vi "AlliGator Update Loaded Dataset Info.vi"(4 "Image Loading Options":T1={"Pixel Well Capacity"=0, "Pile-up Correction"=FALSE, "Gate Step"=0, "Image Smoothing Options"={"Use Image Smoothing"=FALSE, "Kernel Type"=enum."Bilinear", "Bin"=1, "Algorithm"=enum."Rapid"}, "Gates to Skip"={"Start"=0, "End"=0}, "File Background Subtraction"=FALSE, "Background File Path"=path "", "Image Binning Options"={"Use Image Binning"=FALSE, "X Bin"=1, "Y Bin"=1}, "# Gates"=0, "Gates to Keep"={"First"=0, "Last"=0}, "Define Gates to"=FALSE, "Hot Pixel Removal"={"Remove Screamers"=FALSE, "Delta"=0.0, "Equalize Histogram"=FALSE, "Percentile"=0.0, "Hot Pixel Mask Image"=path "", "Use Hot Pixel Mask"=FALSE}, "Dataset Scaling Factor"=0.0, "Image Pre-processing Steps"=[]} {"Hot Pixel Removal"."Percentile" min=0 max=100; "Image Binning Options"."Y Bin" min=1; "Image Binning Options"."X Bin" min=1; "Image Smoothing Options"."Bin" min=1}, 6 "Background File?":bool, 7 "Pile-up Correction":bool, 8 "error in (no error)":errorcluster, 9 "After Loading Dataset Information":T10, 10 "# Gates":i32, 11 "Pixel Well Capacity":u32) -> (0 "Error Out":errorcluster)   [LabVIEW 2021, in "AlliGator Files.lvlib"]
doc: "Updates Settings and Internal Variables after loading a new dataset."
uses:
  AlliGator Files.lvlib
  AlliGator After Loading Dataset Information.ctl
  AlliGator ICCD-specific Information.ctl
  Source Image/AlliGator Image Loading Options.ctl
  Settings/AlliGator Image Smoothing Options.ctl
  Arrays/Kernel Type.ctl
  Arrays/Smoothing Algorithm.ctl
  Settings/AlliGator Background Subtraction Parameters.ctl
  Source Image/AlliGator Image Binning Options.ctl
  Settings/AlliGator Gates to Keep.ctl
  SwissSPAD/SwissSPAD Live_Image Display Options.ctl
  AlliGator Image Pre-processing Step.ctl
  Globals, Variables, Constants/AlliGator Variables List.ctl
  Settings/AlliGator Settings List.ctl
  Globals, Variables, Constants/AlliGator Refnums List.ctl
  Globals, Variables, Constants/AlliGator Globals, Variables & Constants.lvlib
  Settings/AlliGator Settings.lvlib
  GUI/AlliGator GUI.lvlib
  Arrays/Arrays.lvlib
  Source Image/AlliGator Source Image.lvlib
  SwissSPAD/SwissSPAD Live.lvlib
panel:
  # "see the AlliGator License on the block diagram (Ctrl+E or Window:Show Block Diagram)"
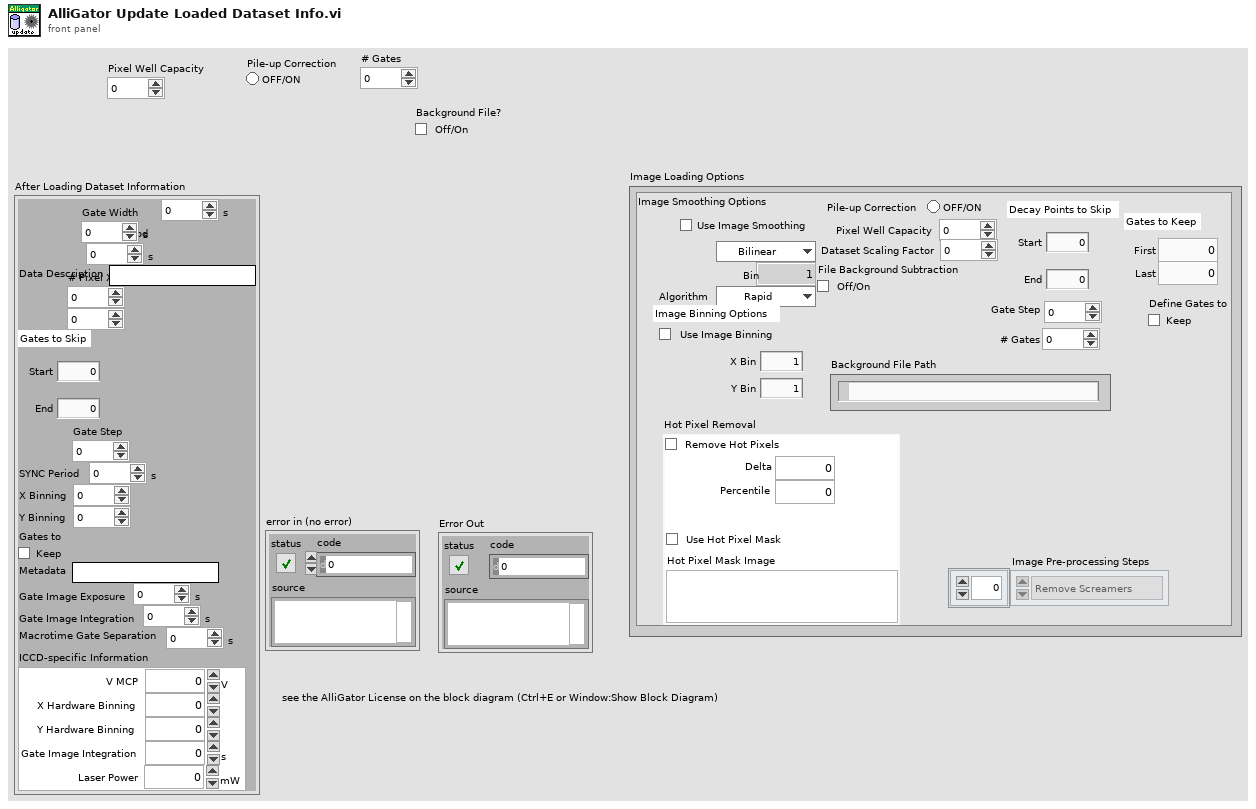
[diagram p1: front panel]
types:
  T1 = typedef "AlliGator Source Image.lvlib/AlliGator Image Loading Options.ctl" = cluster{"Pixel Well Capacity":u32, "Pile-up Correction":bool, "Gate Step":i32, "Image Smoothing Options":T2, "Gates to Skip":T5, "File Background Subtraction":bool, "Background File Path":path, "Image Binning Options":T6, "# Gates":u32, "Gates to Keep":T7, "Define Gates to":bool, "Hot Pixel Removal":T8, "Dataset Scaling Factor":dbl, "Image Pre-processing Steps":T9[]}
  T2 = typedef "AlliGator Settings.lvlib/AlliGator Image Smoothing Options.ctl" = cluster{"Use Image Smoothing":bool, "Kernel Type":T3, "Bin":i32, "Algorithm":T4}
  T3 = typedef "Arrays.lvlib/Kernel Type.ctl" = enum16{"Uniform", "Bilinear", "Gaussian"}
  T4 = typedef "Arrays.lvlib/Smoothing Algorithm.ctl" = enum16{"Rapid", "Thorough"}
  T5 = typedef "AlliGator Settings.lvlib/AlliGator Background Subtraction Parameters.ctl" = cluster{"Start":u32, "End":u32}
  T6 = typedef "AlliGator Source Image.lvlib/AlliGator Image Binning Options.ctl" = cluster{"Use Image Binning":bool, "X Bin":i32, "Y Bin":i32}
  T7 = typedef "AlliGator Settings.lvlib/AlliGator Gates to Keep.ctl" = cluster{"First":u32, "Last":u32}
  T8 = typedef "SwissSPAD Live.lvlib/SwissSPAD Live_Image Display Options.ctl" = cluster{"Remove Screamers":bool, "Delta":sgl, "Equalize Histogram":bool, "Percentile":sgl, "Hot Pixel Mask Image":path, "Use Hot Pixel Mask":bool}
  T9 = typedef "AlliGator Files.lvlib/AlliGator Image Pre-processing Step.ctl" = enum16{"Remove Screamers", "Pile-up Correction", "Binning", "Smoothing", "Rescaling", "Dead Left Column Correction"}
  T10 = typedef "AlliGator Files.lvlib/AlliGator After Loading Dataset Information.ctl" = cluster{"Nanotime Gate Separation":dbl[unit], "Gate Width":dbl[unit], "Laser Period":dbl[unit], "Data Description":string, "# Pixel X":i32, "# Pixel Y":i32, "Gates to Use":cluster{"Start":u32, "End":u32}, "Gate Step":i32, "SYNC Period":dbl[unit], "X Binning":i32, "Y Binning":i32, "Gates to":bool, "Metadata":string, "Gate Image Exposure":dbl[unit], "Gate Image Integration":dbl[unit], "Macrotime Gate Separation":dbl[unit], "ICCD-specific Information":T11}
  T11 = typedef "AlliGator Files.lvlib/AlliGator ICCD-specific Information.ctl" = cluster{"V MCP":dbl[unit], "X Hardware Binning":dbl, "Y Hardware Binning":dbl, "Gate Image Integration":dbl[unit], "Laser Power":dbl[unit]}
  T12 = typedef "AlliGator Globals, Variables & Constants.lvlib/AlliGator Variables List.ctl" = enum16{"---- GUI ----", "GUI:Initialization Status", "GUI:State Indicators Refnum", "GUI:Original AlliGator Menu Items", "GUI:Current Action Loop State", "GUI:Script in progress", "GUI:Playback", "GUI:Loop Playback", "GUI:Search ROI Used", "GUI:Search ROI", "Decay Graph Max Legend Size", "Intensity Graph Max Legend Size", "Decay Statistics Graph Max Legend Size", "Phasor Graph Max Legend Size", "Phasor Ratio Graph Max Legend Size", "Lifetime Graph Max Legend Size", "---- Files ----", "Files:Export Dataset Frames as Individual Files", "Files:Show Batch Export Help Balloons", "Files:Frames in Dataset", "Files:ptu File Frame Start Indices", "Files:Current Frame in Dataset", "Files:Current Frame Timestamp", "Files:Dataset Loaded", "Files:Dataset Metadata", "Files:Dataset Channel", "Files:Dataset Data Description", "Files:Background Dataset Metadata", "Files:Background Dataset Channel", "Files:Background Dataset Data Description", "Files:Background File Subtraction", "Files:Background File Path", "Files:Background File Pile-up Correction", "Files:Background File Pixel Well Capacity", "Files:Background File Scaling Factor", "Files:Current Dataset Load Settings", "Files:Dataset Path", "Files:ICCD-specific Information", "Files:Macrotime Gate Separation", "------ Python Plugins ------", "Python Plugins:Information", "Python Plugins:Python Session", "Python Plugins:Valid Python Session?", "---- Source Image ----", "Source Image:ROIs", "Source Image:Current ROI", "Source Image:ROI Event Refnum", "X_Source Image Display Range", "X_Source Image Palette Information", "X_Type of Displayed Image", "X_Time Gate Slider", "Source Image:Palette List", "Source Image:Scale", "Source Image:ROI Overlay Color", "Source Image:Overlay to Erase", "Source Image:Is Displayed Image Accumulated", "Source Image:White Light Image Modified", "Source Image:Mask Image Modified", "---- Image Profile Window ----", "Image Profile:Window Event Refnum", "Image Profile:IntensityType", "Image Profile:Intensity Average Type", "Image Profile:Intensity-weighted SDV", "Image Profile:Box Profile Type", "Image Profile:Window Open", "Image Profile:Plotted Fit Parameter", "------ Phasor Graph -------", "Phasor Graph:Show Line", "---- Phasor Plot ---", "Phasor Plot:Parameters Changed", "Phasor Plot:FLI Dataset Modified since last Calculation", "Phasor Harmonics Data", "Selected Phasor Harmonics", "Phasor Harmonic Manager Event Refnum", "Phasor Plot:ROIs", "Phasor Plot:Current ROI", "Phasor Plot:ROI Event Refnum", "Phasor Plot:Image Reference Points", "Phasor Plot:Computed", "Phasor Plot:Palette Information", "Phasor Plot:Palette List", "Phasor Plot:Phasor Ratio Palette Information", "Phasor Plot:Phasor Ratio Palette List", "Phasor Plot:Image Scale", "Phasor Plot:Image Overlay to Erase", "Phasor Plot:Image Elements to Update", "Phasor Plot:Current Calculation Parameters", "Phasor Plot:Current Calibration Options", "Phasor Plot:Reset Cumulated Phasor Plot", "Phasor Plot:Reference 1", "Phasor Plot:Lifetime Reference 1", "Phasor Plot:Reference 1 Frequency", "Phasor Plot:Reference 2", "Phasor Plot:Lifetime Reference 2", "Phasor Plot:Reference 2 Frequency", "---- Decay Analysis ----", "Number of Selected Decays to Fit", "LS Fit Results", "LAR Fit Results", "BS Fit Results", "Last Decay Max - Min", "Best Fit Parameters", "Best Fit Parameter Names", "Actual Size X", "Actual Size Y", "Binning X", "Binning Y", "Actual # Gates", "Dataset Number", "Gates to...", "Gates Skipped", "Gates to keep", "Gate Step", "Gate Separation", "Reversed Gates", "Pile-up Correction", "Pixel Well Capacity", "Background Subtracted", "Background Subtraction Method", "Background Definition Range", "Background File (deprecated)", "Number of Dataset Accumulated", "Array of Accumulated Dataset Paths", "Do Averaged Datasets", "Destination File Path", "Process Plot Target", "Use 1/D as Phasor Frequency", "---- Decay Fit Parameter Map -----", "Decay Fit Parameter Map:Palette Information", "Decay Fit Parameter Map:Palette List", "---- Parameter Map ----", "Parameter Map:Palette Information", "Parameter Map:Palette List", "------- Local Decay Window ---------", "Local Decay Graph Window:Event Refnum", "Local Decay Graph Window:Use normalized IRF for convolution", "----- Miscellaneous ----", "Misc:Skippable Dialog Windows Status"}
  T13 = typedef "AlliGator Settings.lvlib/AlliGator Settings List.ctl" = enum16{"GUI:Visible Settings Tab", "GUI:Last Run Version", "Source Image:Use Image Histogram for Contrast", "Source Image:Low Count Pixels Rejection Options", "Source Image:High Count Pixels Rejection Options", "Source Image:Use Image Brightness", "Source Image:Blend Overlay with Image Background", "Source Image:Use Fixed ROI Diameter", "Source Image:ROI Diameter", "Source Image:ROI Center Color", "Source Image:Peak Threshold", "Source Image:Intensity Threshold", "Source Image:Image Binning Options", "Source Image:Image Smoothing Options", "Source Image:Image Histogram Active", "Source Image:Invert Binary Mask", "Source Image:Hot Pixel Removal", "Source Image:Overlay Analyzed ROI Center", "Source Image:Auto-Adjust Contrast", "Source Image:Histogram Lower Percentile", "Source Image:Histogram Upper Percentile", "Source Image:Save Source Image", "Source Image:Scale Bar Options", "Source Image:Image Resolution (Pixel Size)", "Source Image:Flatfield Correction", "Source Image:Show Dead Left Columns Correction", "Source Image:Dead Left Columns Correction", "Source Image:Image Pre-Processing Operations Order", "Source Image:Overlay ROI Median", "Source Image:Median Overlay Color", "Data Information:Gate Width", "Data Information:Nanotime Gate Separation", "Data Information:Macrotime Gate Separation", "Data Information:Gate Step", "Data Information:# Gates", "Data Information:Gate Image Exposure", "Data Information:Gate Image Integration", "Data Information:Gates to Skip", "Data Information:Gates to Keep", "Data Information:Define Gates to", "Data Information:Channel Name", "Data Information:Available Channel Names", "Data Information:Channel Arithmetic", "Data Information:Background File Subtraction", "Data Information:Background File", "Data Information:Background Scaling Factor", "Data Information:Background Pile-up Correction", "Data Information:Background Pixel Well Capacity", "Data Information:Laser Period", "Data Information:SYNC Period", "Data Information:Pile-up Correction", "Data Information:Pixel Well Capacity", "Data Information:Dataset Scaling Factor", "Fluorescence Decay_Decay Pre-Processing:Reverse Gates", "Fluorescence Decay_Decay Pre-Processing:Verbose Decay Pre-Processing", "Fluorescence Decay_Decay Pre-Processing:Use Decay Pre-Processing", "Fluorescence Decay_Decay Pre-Processing:Background Subtraction", "Fluorescence Decay_Decay Pre-Processing:Background Definition Range", "Fluorescence Decay_Decay Pre-Processing:Baseline Subtraction Method", "Fluorescence Decay_Decay Pre-Processing:Decay Pre-Processing Operations Order", "Fluorescence Decay_Decay Pre-Processing:Smoothing Parameter", "Fluorescence Decay_Decay Pre-Processing:Shift Decay", "Fluorescence Decay_Decay Pre-Processing:Decay Shift Parameters", "Fluorescence Decay_Decay Pre-Processing:Fold Decay", "Fluorescence Decay_Decay Pre-Processing:# Folds", "Fluorescence Decay_Decay Pre-Processing:1-Normalize Decay", "Fluorescence Decay_Decay Pre-Processing:[0-1]-Normalize Decay", "Fluorescence Decay_Decay Pre-Processing:Smoothen Decay", "Fluorescence Decay_Decay Pre-Processing:Extrapolate Decay", "Fluorescence Decay_Decay Pre-Processing:Use Periodicity", "Fluorescence Decay_Decay Pre-Processing:Use Cursors", "Fluorescence Decay_Decay Pre-Processing:Tail Fraction", "Fluorescence Decay_Decay Pre-Processing:Head Fraction", "Fluorescence Decay_Decay Pre-Processing:Additional Points", "Fluorescence Decay_Decay Pre-Processing:Straighten Decay", "Fluorescence Decay_Decay Pre-Processing:Constant Background", "Fluorescence Decay_Decay Pre-Processing:Pixel-Normalize Decay", "Fluorescence Decay_Advanced Analysis:Extract IRF instead of Decay", "Fluorescence Decay_Advanced Analysis:IRF Extraction Options", "Fluorescence Decay_Advanced Analysis:IRF Optimization Options", "Fluorescence Decay_Advanced Analysis:Square Pulse Options", "Fluorescence Decay_Advanced Analysis:IRF Order", "Fluorescence Decay_Advanced Analysis:IRF Time Constants", "Fluorescence Decay_Advanced Analysis:Wavelet Analysis Options", "Fluorescence Decay_Advanced Analysis:Average Lifetime Options", "Fluorescence Decay_Fit Options:Fit Options", "Fluorescence Decay_Fit Options:Use Legacy Fitting Approach", "Fluorescence Decay_Fit Options:Use Data Information Laser Period", "Fluorescence Decay_Fit Parameters:Displayed Fit Parameters", "Fluorescence Decay_Fit Parameters:Fit Parameter Constraints", "Fluorescence Decay_Fit Parameters:Export Tabulated Results", "Fluorescence Decay_Fit Parameters:MLE Baseline Offset Type", "Fluorescence Decay_Fit Parameters:MLE Baseline Offset", "Fluorescence Decay_Fit Parameters:Guess Parameter Names", "Fluorescence Decay_Fit Parameters:Guess Parameter Values", "Fluorescence Decay_Fit Parameters:Guess Parameters Options", "Fluorescence Decay_Styles:Show Last Decay Only", "Fluorescence Decay_Styles:Decay Graph Color Array", "Fluorescence Decay:Decay Graph Active", "Fluorescence Decay Statistics:Min Peak Value", "Fluorescence Decay Statistics:Reject Low Decay Peak Pixels", "Fluorescence Decay Statistics:Reject High Decay Peak Pixels", "Fluorescence Decay Statistics:Max Peak Value", "Time Traces:Use File Timestamp", "Time Traces:Time Step", "Time Traces:Use Intensity Correction File", "Time Traces:Intensity Correction File", "Phasor Plot:Phasor Plot Smoothing Options", "Phasor Plot:Phasor Plot Size", "Phasor Plot:Phasor Plot Graphics Options", "Phasor Plot:Cumulative Phasor Plot", "Phasor Plot:Use Phasor Brightness", "Phasor Plot:Blend Overlay with Phasor Background", "Phasor Plot:Save Phasor Plot", "Phasor Plot:Show References", "Phasor Plot:Phasor Ratio Decay Range", "Phasor Plot:Exponential Fading", "Phasor Plot:Phasor Ratio Reference Colors", "Phasor Plot:Reference Radius", "Phasor Plot:Show Color Map Vertices", "Phasor Plot:Phasor Plot Active", "Phasor Plot:Phasor Ratio Color Map Type", "Phasor Plot:Phasor Ratio Color Map", "Phasor Plot:Phasor Ratio Display Range", "Phasor Plot:Selected Image ROI(s)", "Phasor Plot:All Image ROIs", "Phasor Plot:Selected Phasor Plot ROI(s)", "Phasor Plot:All Phasor Plot ROIs", "Phasor Plot:Phasor Ratio Color-Coded Quantity", "Phasor Plot:Store Phasor Harmonics", "Phasor Plot:Draw Reference Segment", "Phasor Plot:User-Defined Quantity", "Phasor Graph:Phasor Frequency", "Phasor Graph:Phasor Ratio Type", "Phasor Graph:Pixel-level Phasor Computation", "Phasor Graph:Save Phasor Graph", "Phasor Graph:Phasor Graph Active", "Phasor Graph:Phasor SDV Options", "Phasor Calibration:Use Backup Calibration if needed", "Phasor Graph:Define Shortest Lifetime as", "Phasor Calibration:Backup Calibration Type", "Phasor Calibration:Calibration Type", "Phasor Calibration:Calibration Lifetime", "Phasor Calibration:Calibration Map Algorithm", "Single-Exponential Phasor Locus (SEPL):Gate Parameters", "Single-Exponential Phasor Locus (SEPL):User-defined Gate", "Single-Exponential Phasor Locus (SEPL):User-defined IRF", "Single-Exponential Phasor Locus (SEPL):Phasor Parameters", "Single-Exponential Phasor Locus (SEPL):Decay & IRF Parameters", "Single-Exponential Phasor Locus (SEPL):Display Parameters", "Lifetime Analysis:Decay Analysis Parameters", "Lifetime Analysis:Lifetime Map Active", "Plugins:Python Settings", "Miscellaneous:Verbose Mode", "Miscellaneous:Beep after Script", "Miscellaneous:Saved Image File Format", "Miscellaneous:Exported Gate Image Settings", "Miscellaneous:Include Loading in Timing", "Miscellaneous:Verbose Settings Mode", "Miscellaneous:Histogram Options", "Miscellaneous:Beep on Error", "Miscellaneous:# Logical Processors Used", "Miscellaneous:ROI Description Max Characters", "Miscellaneous:Verbose Error Mode", "Miscellaneous:Transparent Mask Color"}
  T14 = typedef "AlliGator Globals, Variables & Constants.lvlib/AlliGator Refnums List.ctl" = enum16{"---------- AlliGator Controls ----------", "AlliGator Tab Control Refnum", "---------- AlliGator Indicators ----------", "Source Image Display Refnum", "Phasor Plot Display Refnum", "Decay Fit Parameter Map Refnum", "---------- AlliGator VIs ----------", "AlliGator Settings Refnum", "AlliGator Launcher Refnum"}
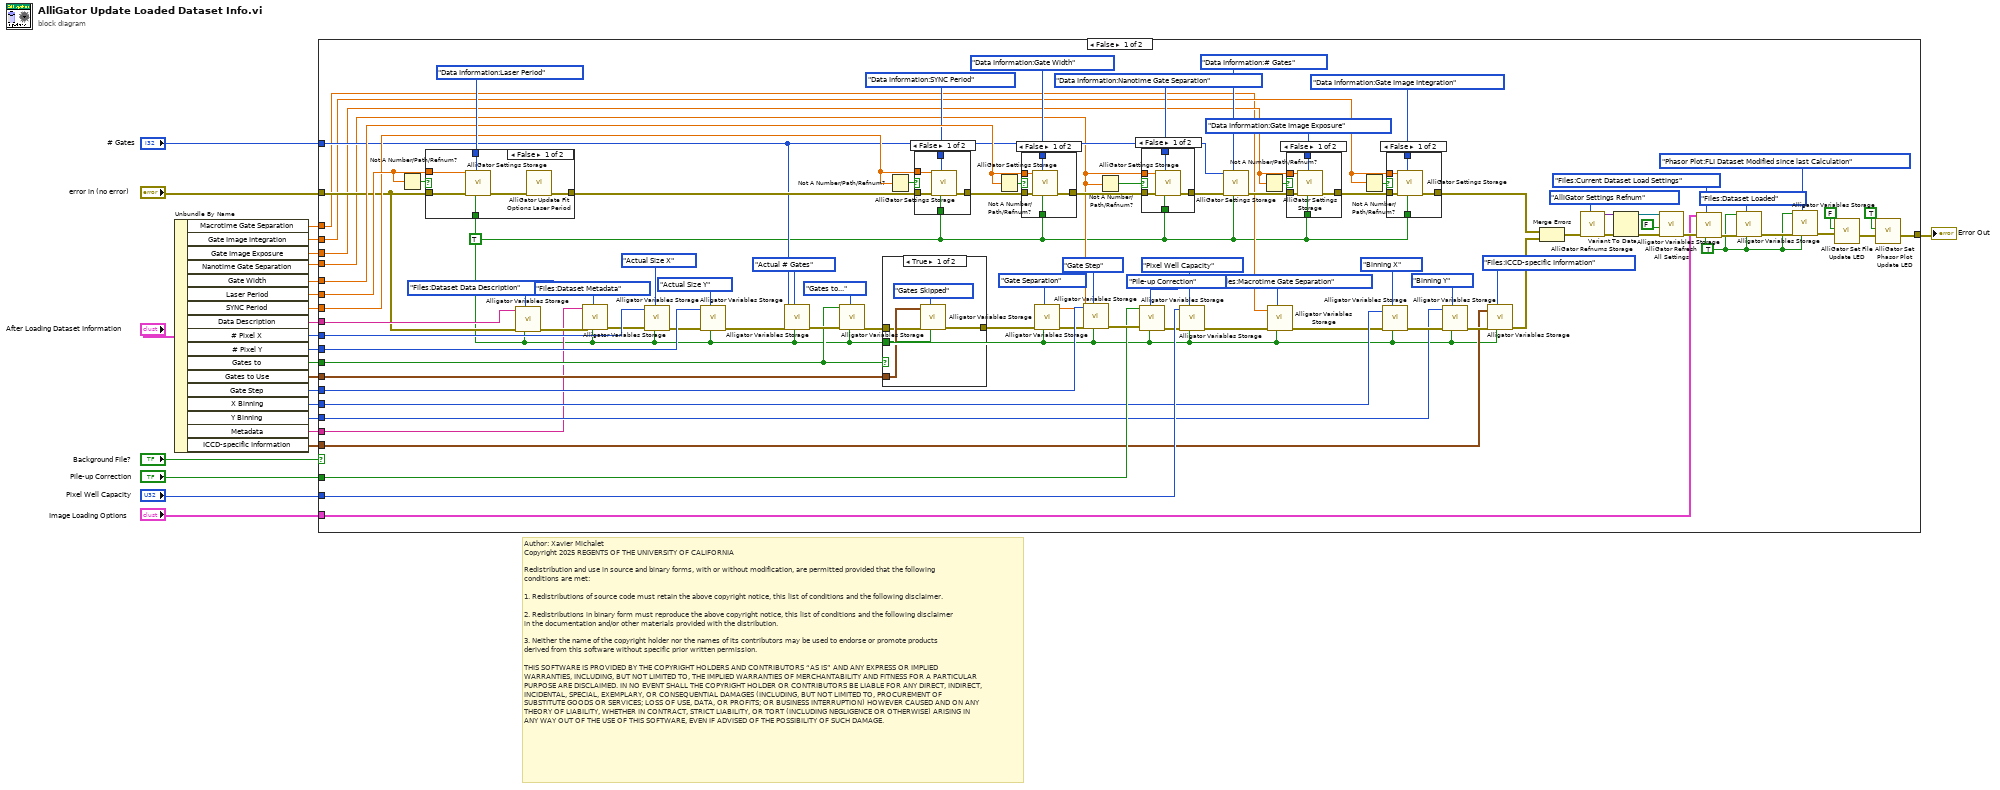
[diagram p0: block diagram]
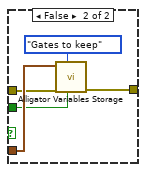
[diagram p6: hidden frame]
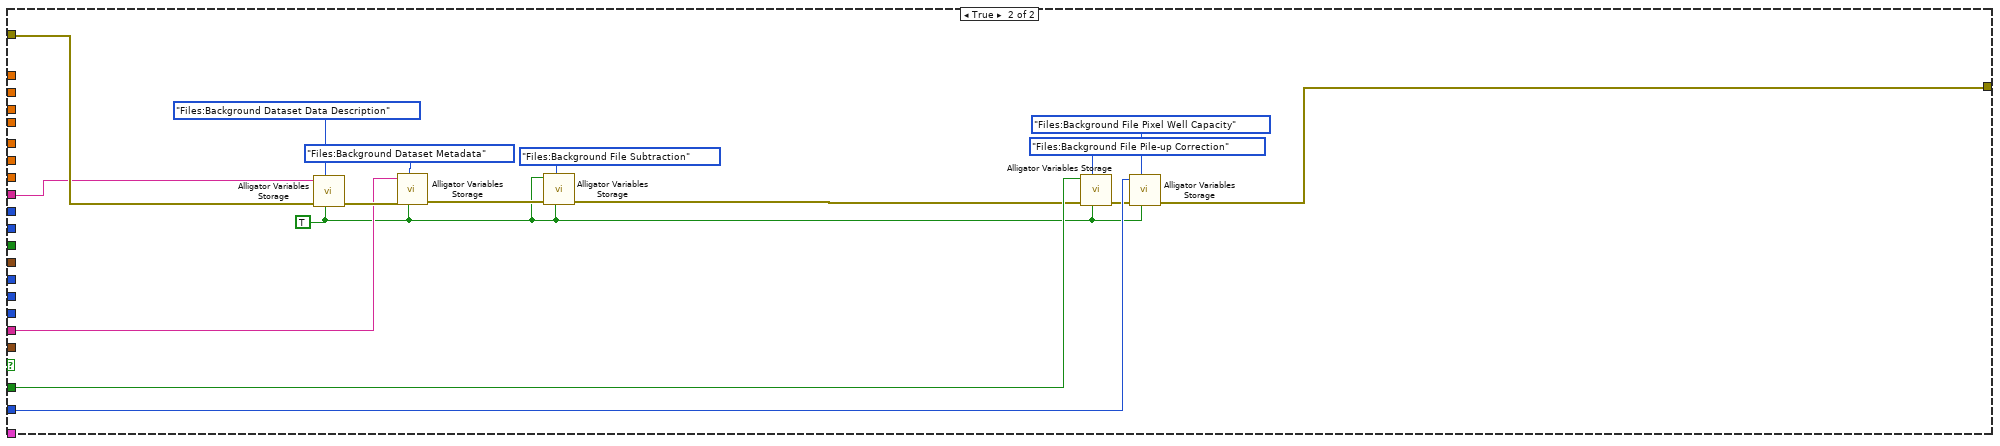
[diagram p9: hidden frame]
diagram:
  # "Author: Xavier Michalet\nCopyright 2025 REGENTS OF THE UNIVERSITY OF CALIFORNIA\n\nRedistribution and use in source and binary forms, with or without modification, are permitted provided that the following conditions are met:\n\n1. Redistributions of source code must retain the above copyright notice, this list of conditions and the following disclaimer.\n\n2. Redistributions in binary form must reproduce the above copyright notice, this list of conditions and the following disclaimer in the documentation and/or other materials provided with the distribution.\n\n3. Neither the name of the copyright holder nor the names of its contributors may be used to endorse or promote products derived from this software without specific prior written permission.\n\nTHIS SOFTWARE IS PROVIDED BY THE COPYRIGHT HOLDERS AND CONTRIBUTORS “AS IS” AND ANY EXPRESS OR IMPLIED WARRANTIES, INCLUDING, BUT NOT LIMITED TO, THE IMPLIED WARRANTIES OF MERCHANTABILITY AND FITNESS FOR A PARTICULAR PURPOSE ARE DISCLAIMED. IN NO EVENT SHALL THE COPYRIGHT HOLDER OR CONTRIBUTORS BE LIABLE FOR ANY DIRECT, INDIRECT, INCIDENTAL, SPECIAL, EXEMPLARY, OR CONSEQUENTIAL DAMAGES (INCLUDING, BUT NOT LIMITED TO, PROCUREMENT OF SUBSTITUTE GOODS OR SERVICES; LOSS OF USE, DATA, OR PROFITS; OR BUSINESS INTERRUPTION) HOWEVER CAUSED AND ON ANY THEORY OF LIABILITY, WHETHER IN CONTRACT, STRICT LIABILITY, OR TORT (INCLUDING NEGLIGENCE OR OTHERWISE) ARISING IN ANY WAY OUT OF THE USE OF THIS SOFTWARE, EVEN IF ADVISED OF THE POSSIBILITY OF SUCH DAMAGE."
  n1 = Unbundle By Name("After Loading Dataset Information") -> ("Macrotime Gate Separation"=w2:dbl[unit], "Gate Image Integration"=w3:dbl[unit], "Gate Image Exposure"=w4:dbl[unit], "Nanotime Gate Separation"=w9:dbl[unit], "Gate Width"=w18:dbl[unit], "Laser Period"=w19:dbl[unit], "SYNC Period"=w16:dbl[unit], "Data Description"=w11:string, "# Pixel X"=w23:i32, "# Pixel Y"=w24:i32, "Gates to"=w12:bool, "Gates to Use"=w25:cluster{"Start":u32, "End":u32}, "Gate Step"=w15:i32, "X Binning"=w14:i32, "Y Binning"=w13:i32, "Metadata"=w5:string, "ICCD-specific Information"=w1:T11)
  n2 = case shown="False" "Background File?" {
    tunnel: w25 -> [w116 _]
    tunnel: w24 -> [w115 _]
    tunnel: w23 -> [w114 _]
    tunnel: "Pile-up Correction" -> [w110 w179]
    tunnel: "Pixel Well Capacity" -> [w109 w178]
    tunnel: w19 -> [w99 _]
    tunnel: w18 -> [w97 _]
    tunnel: "# Gates" -> [w45 _]
    tunnel: w16 -> [w89 _]
    tunnel: w15 -> [w85 _]
    tunnel: w14 -> [w81 _]
    tunnel: w13 -> [w80 _]
    tunnel: w12 -> [w69 _]
    tunnel: w11 -> [w68 w171]
    tunnel: "error in (no error)" -> [w66 w172]
    tunnel: w9 -> [w36 _]
    tunnel: [w58 w177] -> w7
    tunnel: "Image Loading Options" -> [w53 _]
    tunnel: w5 -> [w49 w173]
    tunnel: w4 -> [w38 _]
    tunnel: w3 -> [w37 _]
    tunnel: w2 -> [w32 _]
    tunnel: w1 -> [w28 _]
    frame False {
      w54 = TRUE ("Get(F)/Set")
      w26 = TRUE ("Get(F)/Set")
      n3 = Not A Number/Path/Refnum?(number/path/refnum=w99) -> (NaN/Path/Refnum?=w98:bool)
      n4 = case shown="False" w98 {
        tunnel: w26 -> [w162 _]
        tunnel: [w158 w163] -> w92
        tunnel: AlliGator_Settings_List."Data Information:Laser Period" ("AlliGator Settings List") -> [w161 _]
        tunnel: w99 -> [w157 _]
        tunnel: w66 -> [w160 w163]
        frame False {
          n5 = call "AlliGator Settings Storage.vi"("Get(F)/Set"=w162, "AlliGator Settings List"=w161, "Error In"=w160, "Variant Data in"=w157) -> ("Error Out"=w159:errorcluster)  [unwired: 6 in, 1 out]
          n6 = call "AlliGator Update Fit Options Laser Period.vi"("error in (no error)"=w159) -> ("error out"=w158:errorcluster)  [unwired: 10 in]
        }
        frame True {
        }
      }
      n7 = call "Alligator Variables Storage.vi"("Get(F)/Set"=w26, "AlliGator Variable"=AlliGator_Variables_List."Files:Dataset Data Description" ("Alligator Variable"), "Error In"=w66, "Data in"=w68) -> ("Error Out"=w52:errorcluster)  [unwired: 5 in, 2 out]
      n8 = call "Alligator Variables Storage.vi"("Get(F)/Set"=w26, "AlliGator Variable"=AlliGator_Variables_List."Files:Dataset Metadata" ("Alligator Variable"), "Error In"=w52, "Data in"=w49) -> ("Error Out"=w51:errorcluster)  [unwired: 5 in, 2 out]
      n9 = call "Alligator Variables Storage.vi"("Get(F)/Set"=w26, "AlliGator Variable"=AlliGator_Variables_List."Actual Size X" ("Alligator Variable"), "Error In"=w51, "Data in"=w114) -> ("Error Out"=w105:errorcluster)  [unwired: 5 in, 2 out]
      n10 = call "Alligator Variables Storage.vi"("Get(F)/Set"=w26, "AlliGator Variable"=AlliGator_Variables_List."Actual Size Y" ("Alligator Variable"), "Error In"=w105, "Data in"=w115) -> ("Error Out"=w107:errorcluster)  [unwired: 5 in, 2 out]
      n11 = call "Alligator Variables Storage.vi"("Get(F)/Set"=w26, "AlliGator Variable"=AlliGator_Variables_List."Actual # Gates" ("Alligator Variable"), "Error In"=w107, "Data in"=w45) -> ("Error Out"=w72:errorcluster)  [unwired: 5 in, 2 out]
      n12 = call "Alligator Variables Storage.vi"("Get(F)/Set"=w26, "AlliGator Variable"=AlliGator_Variables_List."Gates to..." ("Alligator Variable"), "Error In"=w72, "Data in"=w69) -> ("Error Out"=w71:errorcluster)  [unwired: 5 in, 2 out]
      n13 = case shown="True" w69 {
        tunnel: w116 -> [w145 w150]
        tunnel: [w143 w148] -> w87
        tunnel: w71 -> [w142 w147]
        tunnel: w26 -> [w141 w146]
        frame True {
          n14 = call "Alligator Variables Storage.vi"("Get(F)/Set"=w141, "AlliGator Variable"=AlliGator_Variables_List."Gates Skipped" ("Alligator Variable"), "Error In"=w142, "Data in"=w145) -> ("Error Out"=w143:errorcluster)  [unwired: 5 in, 2 out]
        }
        frame False {
          n15 = call "Alligator Variables Storage.vi"("Get(F)/Set"=w146, "AlliGator Variable"=AlliGator_Variables_List."Gates to keep" ("Alligator Variable"), "Error In"=w147, "Data in"=w150) -> ("Error Out"=w148:errorcluster)  [unwired: 5 in, 2 out]
        }
      }
      n16 = Not A Number/Path/Refnum?(number/path/refnum=w89) -> (NaN/Path/Refnum?=w90:bool)
      n17 = case shown="False" w90 {
        tunnel: w26 -> [w155 _]
        tunnel: [w154 w156] -> w91
        tunnel: AlliGator_Settings_List."Data Information:SYNC Period" ("AlliGator Settings List") -> [w153 _]
        tunnel: w89 -> [w152 _]
        tunnel: w92 -> [w151 w156]
        frame False {
          n18 = call "AlliGator Settings Storage.vi"("Get(F)/Set"=w155, "AlliGator Settings List"=w153, "Error In"=w151, "Variant Data in"=w152) -> ("Error Out"=w154:errorcluster)  [unwired: 6 in, 1 out]
        }
        frame True {
        }
      }
      n19 = Not A Number/Path/Refnum?(number/path/refnum=w97) -> (NaN/Path/Refnum?=w96:bool)
      n20 = case shown="False" w96 {
        tunnel: w26 -> [w139 _]
        tunnel: [w138 w140] -> w111
        tunnel: AlliGator_Settings_List."Data Information:Gate Width" ("AlliGator Settings List") -> [w137 _]
        tunnel: w91 -> [w136 w140]
        tunnel: w97 -> [w135 _]
        frame False {
          n21 = call "AlliGator Settings Storage.vi"("Get(F)/Set"=w139, "AlliGator Settings List"=w137, "Error In"=w136, "Variant Data in"=w135) -> ("Error Out"=w138:errorcluster)  [unwired: 6 in, 1 out]
        }
        frame True {
        }
      }
      n22 = call "Alligator Variables Storage.vi"("Get(F)/Set"=w26, "AlliGator Variable"=AlliGator_Variables_List."Gate Separation" ("Alligator Variable"), "Error In"=w87, "Data in"=w36) -> ("Error Out"=w73:errorcluster)  [unwired: 5 in, 2 out]
      n23 = call "Alligator Variables Storage.vi"("Get(F)/Set"=w26, "AlliGator Variable"=AlliGator_Variables_List."Gate Step" ("Alligator Variable"), "Error In"=w73, "Data in"=w85) -> ("Error Out"=w112:errorcluster)  [unwired: 5 in, 2 out]
      n24 = Not A Number/Path/Refnum?(number/path/refnum=w36) -> (NaN/Path/Refnum?=w95:bool)
      n25 = call "Alligator Variables Storage.vi"("Get(F)/Set"=w26, "AlliGator Variable"=AlliGator_Variables_List."Pile-up Correction" ("Alligator Variable"), "Error In"=w112, "Data in"=w110) -> ("Error Out"=w46:errorcluster)  [unwired: 5 in, 2 out]
      n26 = case shown="False" w95 {
        tunnel: [w133 w134] -> w93
        tunnel: w26 -> [w132 _]
        tunnel: w111 -> [w131 w134]
        tunnel: AlliGator_Settings_List."Data Information:Nanotime Gate Separation" ("AlliGator Settings List") -> [w130 _]
        tunnel: w36 -> [w129 _]
        frame False {
          n27 = call "AlliGator Settings Storage.vi"("Get(F)/Set"=w132, "AlliGator Settings List"=w130, "Error In"=w131, "Variant Data in"=w129) -> ("Error Out"=w133:errorcluster)  [unwired: 6 in, 1 out]
        }
        frame True {
        }
      }
      n28 = call "Alligator Variables Storage.vi"("Get(F)/Set"=w26, "AlliGator Variable"=AlliGator_Variables_List."Pixel Well Capacity" ("Alligator Variable"), "Error In"=w46, "Data in"=w109) -> ("Error Out"=w34:errorcluster)  [unwired: 5 in, 2 out]
      n29 = call "AlliGator Settings Storage.vi"("Get(F)/Set"=w26, "AlliGator Settings List"=AlliGator_Settings_List."Data Information:# Gates", "Error In"=w93, "Variant Data in"=w45) -> ("Error Out"=w42:errorcluster)  [unwired: 6 in, 1 out]
      n30 = Not A Number/Path/Refnum?(number/path/refnum=w38) -> (NaN/Path/Refnum?=w44:bool)
      n31 = call "Alligator Variables Storage.vi"("Get(F)/Set"=w26, "AlliGator Variable"=AlliGator_Variables_List."Files:Macrotime Gate Separation" ("Alligator Variable"), "Error In"=w34, "Data in"=w32) -> ("Error Out"=w33:errorcluster)  [unwired: 5 in, 2 out]
      n32 = case shown="False" w44 {
        tunnel: w26 -> [w127 _]
        tunnel: [w126 w128] -> w41
        tunnel: AlliGator_Settings_List."Data Information:Gate Image Exposure" ("AlliGator Settings List") -> [w125 _]
        tunnel: w42 -> [w124 w128]
        tunnel: w38 -> [w123 _]
        frame False {
          n33 = call "AlliGator Settings Storage.vi"("Get(F)/Set"=w127, "AlliGator Settings List"=w125, "Error In"=w124, "Variant Data in"=w123) -> ("Error Out"=w126:errorcluster)  [unwired: 6 in, 1 out]
        }
        frame True {
        }
      }
      n34 = Not A Number/Path/Refnum?(number/path/refnum=w37) -> (NaN/Path/Refnum?=w43:bool)
      n35 = call "Alligator Variables Storage.vi"("Get(F)/Set"=w26, "AlliGator Variable"=AlliGator_Variables_List."Binning X" ("Alligator Variable"), "Error In"=w33, "Data in"=w81) -> ("Error Out"=w84:errorcluster)  [unwired: 5 in, 2 out]
      n36 = case shown="False" w43 {
        tunnel: w26 -> [w121 _]
        tunnel: [w120 w122] -> w35
        tunnel: AlliGator_Settings_List."Data Information:Gate Image Integration" ("AlliGator Settings List") -> [w119 _]
        tunnel: w41 -> [w118 w122]
        tunnel: w37 -> [w117 _]
        frame False {
          n37 = call "AlliGator Settings Storage.vi"("Get(F)/Set"=w121, "AlliGator Settings List"=w119, "Error In"=w118, "Variant Data in"=w117) -> ("Error Out"=w120:errorcluster)  [unwired: 6 in, 1 out]
        }
        frame True {
        }
      }
      n38 = call "Alligator Variables Storage.vi"("Get(F)/Set"=w26, "AlliGator Variable"=AlliGator_Variables_List."Binning Y" ("Alligator Variable"), "Error In"=w84, "Data in"=w80) -> ("Error Out"=w30:errorcluster)  [unwired: 5 in, 2 out]
      n39 = call "Alligator Variables Storage.vi"("Get(F)/Set"=w26, "AlliGator Variable"=AlliGator_Variables_List."Files:ICCD-specific Information", "Error In"=w30, "Data in"=w28) -> ("Error Out"=w29:errorcluster)  [unwired: 5 in, 2 out]
      n40 = Merge Errors(w35, w29) -> (w76:errorcluster)
      n41 = call "AlliGator Refnums Storage.vi"("AlliGator Refnum List"=AlliGator_Refnums_List."AlliGator Settings Refnum", "Error In"=w76) -> ("Error Out"=w78:errorcluster, "Data out"=w77:variant)  [unwired: 8 in]
      n42 = Variant To Data(error in=w78, Variant=w77) -> (data=w74:refnum<vi>, error out=w75:errorcluster)  [unwired: 1 in]
      n43 = call "AlliGator Refresh All Settings.vi"("Error In"=w75, "Verbose (T)"=FALSE, "VI Refnum in"=w74) -> ("Error Out"=w60:errorcluster)  [unwired: 8 in]
      n44 = call "Alligator Variables Storage.vi"("Get(F)/Set"=w54, "AlliGator Variable"=AlliGator_Variables_List."Files:Current Dataset Load Settings" ("Alligator Variable"), "Error In"=w60, "Data in"=w53) -> ("Error Out"=w64:errorcluster)  [unwired: 5 in, 2 out]
      n45 = call "Alligator Variables Storage.vi"("Get(F)/Set"=w54, "AlliGator Variable"=AlliGator_Variables_List."Files:Dataset Loaded" ("Alligator Variable"), "Error In"=w64, "Data in"=w54) -> ("Error Out"=w57:errorcluster)  [unwired: 5 in, 2 out]
      n46 = call "Alligator Variables Storage.vi"("Get(F)/Set"=w54, "AlliGator Variable"=AlliGator_Variables_List."Phasor Plot:FLI Dataset Modified since last Calculation" ("Alligator Variable"), "Error In"=w57, "Data in"=w54) -> ("Error Out"=w56:errorcluster)  [unwired: 5 in, 2 out]
      n47 = call "AlliGator Set File Update LED.vi"("error in (no error)"=w56, "Off/On"=FALSE) -> ("error out"=w62:errorcluster)  [unwired: 9 in]
      n48 = call "AlliGator Set Phasor Plot Update LED.vi"("error in (no error)"=w62, "Off/On"=TRUE) -> ("error out"=w58:errorcluster)  [unwired: 9 in]
    }
    frame True {
      w164 = TRUE ("Get(F)/Set")
      n49 = call "Alligator Variables Storage.vi"("Get(F)/Set"=w164, "AlliGator Variable"=AlliGator_Variables_List."Files:Background Dataset Data Description" ("Alligator Variable"), "Error In"=w172, "Data in"=w171) -> ("Error Out"=w175:errorcluster)  [unwired: 5 in, 2 out]
      n50 = call "Alligator Variables Storage.vi"("Get(F)/Set"=w164, "AlliGator Variable"=AlliGator_Variables_List."Files:Background Dataset Metadata" ("Alligator Variable"), "Error In"=w175, "Data in"=w173) -> ("Error Out"=w167:errorcluster)  [unwired: 5 in, 2 out]
      n51 = call "Alligator Variables Storage.vi"("Get(F)/Set"=w164, "AlliGator Variable"=AlliGator_Variables_List."Files:Background File Subtraction" ("Alligator Variable"), "Error In"=w167, "Data in"=w164) -> ("Error Out"=w166:errorcluster)  [unwired: 5 in, 2 out]
      n52 = call "Alligator Variables Storage.vi"("Get(F)/Set"=w164, "AlliGator Variable"=AlliGator_Variables_List."Files:Background File Pile-up Correction" ("Alligator Variable"), "Error In"=w166, "Data in"=w179) -> ("Error Out"=w168:errorcluster)  [unwired: 5 in, 2 out]
      n53 = call "Alligator Variables Storage.vi"("Get(F)/Set"=w164, "AlliGator Variable"=AlliGator_Variables_List."Files:Background File Pixel Well Capacity" ("Alligator Variable"), "Error In"=w168, "Data in"=w178) -> ("Error Out"=w177:errorcluster)  [unwired: 5 in, 2 out]
    }
  }
  "Error Out" <- w7
